vi "Initialize.vi"(8 "error in (no error)":errorcluster, 10 "Serial Config":T1 {"Parity" items=["None", "Odd", "Even"]; "Flow Ctl" items=["None"]; "Baud" items=["4800"=4800, "9600"=9600, "19200"=19200, "38400"=38400]}, 11 "VISA resource in":refnum<visa-resource-name>) -> (0 "error out":errorcluster, 2 "read buffer":string, 3 "VISA resource out":refnum<visa-resource-name>)   [LabVIEW 2014, in "B&K Precision 9120 series.lvclass"]
uses:
  B&K Precision 9120 series.lvclass
  Serial_Config.ctl
  <vilib>/Instr/_visa.llb/VISA Set IO Buffer Mask.ctl
  <vilib>/Utility/error.llb/Error Cluster From Error Code.vi
  <vilib>/ErrorRing/Error Ring.xnode
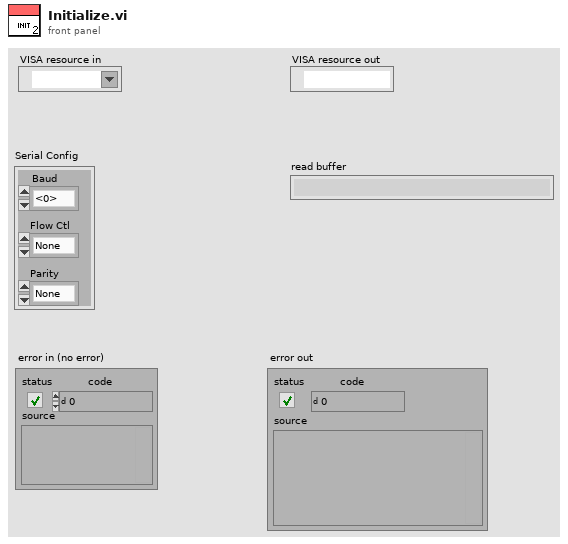
[diagram p1: front panel]
types:
  T1 = typedef "B&K Precision 9120 series.lvclass/Serial_Config.ctl" = cluster{"Baud":u32, "Flow Ctl":u16, "Parity":u16}
  T2 = typedef "VISA Set IO Buffer Mask.ctl" = u16
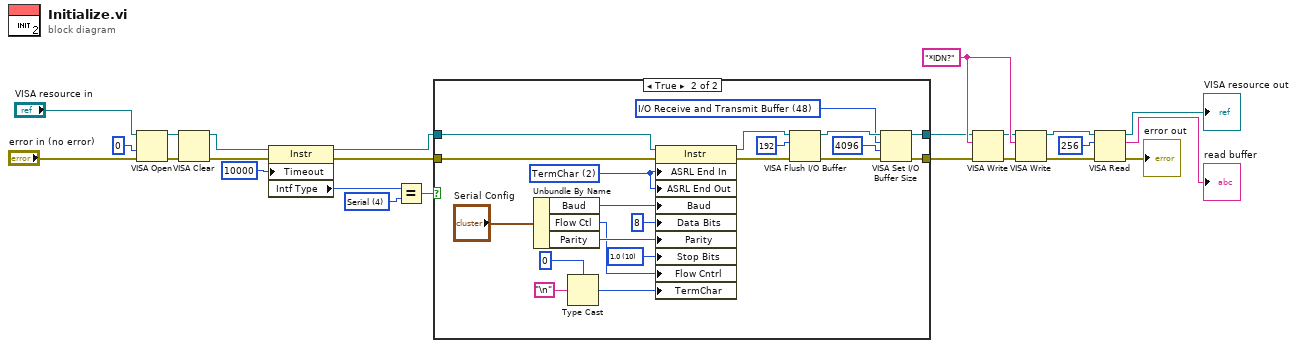
[diagram p0: block diagram]
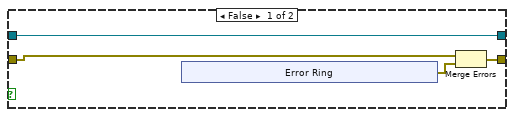
[diagram p2: hidden frame]
diagram:
  w8 = "*IDN?" ("write buffer")
  w15 = u16 4 items=["GPIB"=1, "VXI"=2, "GPIB-VXI"=3, "Serial"=4, "PXI"=5, "TCPIP"=6, "USB"=7] ("Interface Information:Interface Type")
  n1 = VISA Open(access mode=0, error in (no error)="error in (no error)", VISA resource name="VISA resource in") -> (VISA resource name=w20:refnum<visa-resource-name>, error out=w21:errorcluster)  [unwired: 2 in]
  n2 = VISA Clear(VISA resource name=w20, error in (no error)=w21) -> (VISA resource name out=w19:refnum<visa-resource-name>, error out=w18:errorcluster)
  n3 = property class="Instr"(reference=w19, error in=w18, "Timeout"=u32 10000 ("General Settings:Timeout Value")) -> (reference out=w13:refnum<visa-resource-name>, error out=w12:errorcluster, "Intf Type"=w16:u16)
  n4 = Equal?(x=w16, y=w15) -> (x = y?=w14:bool)
  n5 = case shown="True" w14 {
    tunnel: w13 -> [w28 w53]
    tunnel: w12 -> [w25 w52]
    tunnel: [w28 w34] -> w5
    tunnel: [w26 w33] -> w4
    frame False {
      n6 = xnode "Error Ring"() -> ("error out"=w27:errorcluster)
      n7 = Merge Errors(w25, w27) -> (w26:errorcluster)
    }
    frame True {
      w36 = T2 48 items=["I/O Receive Buffer"=16, "I/O Transmit Buffer"=32, "I/O Receive and Transmit Buffer"=48] ("Mask")
      w42 = u16 2 items=["None", "Last Bit", "TermChar", "Break"] ("Serial Settings:End Mode for Writes")
      w48 = u16 10 items=["1.0"=10, "1.5"=15, "2.0"=20] ("Serial Settings:Stop Bits")
      n8 = Unbundle By Name("Serial Config") -> ("Baud"=w43:u32, "Flow Ctl"=w47:u16, "Parity"=w49:u16)
      n9 = Type Cast(type=u8 0, x="\n") -> (*(type *) &x=w44:u8)
      n10 = property class="Instr"(reference=w53, error in=w52, "ASRL End In"=w42, "ASRL End Out"=w42, "Baud"=w43, "Data Bits"=u16 8 ("Serial Settings:Data Bits"), "Parity"=w49, "Stop Bits"=w48, "Flow Cntrl"=w47, "TermChar"=w44) -> (reference out=w41:refnum<visa-resource-name>, error out=w40:errorcluster)
      n11 = VISA Flush I/O Buffer(VISA resource name=w41, mask (16)=192, error in (no error)=w40) -> (VISA resource name out=w38:refnum<visa-resource-name>, error out=w37:errorcluster)
      n12 = VISA Set I/O Buffer Size(VISA resource name=w38, mask (16)=w36, size (4096)=u32 4096, error in (no error)=w37) -> (VISA resource name out=w34:refnum<visa-resource-name>, error out=w33:errorcluster)
    }
  }
  n13 = VISA Write(VISA resource name=w5, write buffer=w8, error in (no error)=w4) -> (VISA resource name out=w6:refnum<visa-resource-name>, error out=w7:errorcluster)  [unwired: 1 out]
  n14 = VISA Write(VISA resource name=w6, write buffer=w8, error in (no error)=w7) -> (VISA resource name out=w10:refnum<visa-resource-name>, error out=w9:errorcluster)  [unwired: 1 out]
  n15 = VISA Read(VISA resource name=w10, byte count=u32 256, error in (no error)=w9) -> (VISA resource name out=→"VISA resource out":refnum<visa-resource-name>, read buffer=→"read buffer":string, error out=→"error out":errorcluster)  [unwired: 1 out]
